vi "PCA9525 - 24V.vi"(8 "error in (no error)":errorcluster, 11 "handle":u64 format="%x") -> (0 "error out":errorcluster, 2 "buffer":u8[](array[numeric]), 3 "handle 2":u64)   [LabVIEW 2024]
uses:
  I2C/libmpsse.dll
  I2C/libMPSSE-I2C.lvlib
panel:
  out "sizeTransferred 2":u32
  out "p/f4":bool
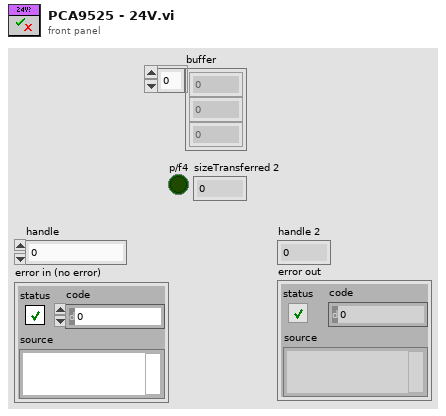
[diagram p1: front panel]
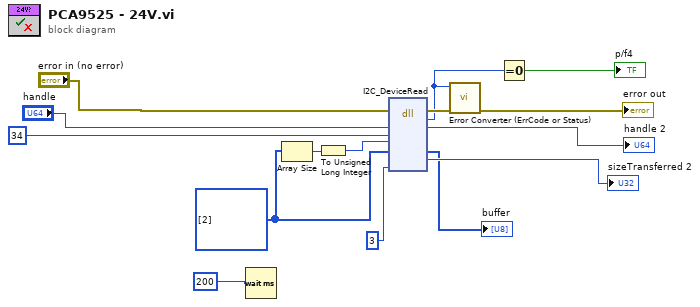
[diagram p0: block diagram]
diagram:
  w7 = u8[] [2] ("*buffer 3")
  n1 = Wait (ms)(milliseconds to wait=u32 200) -> ()  [unwired: 1 out]
  n2 = Array Size(array=w7) -> (size(s)=w6:i32)
  n3 = To Unsigned Long Integer(number=w6) -> (unsigned 32bit integer=w8:u32)
  n4 = dll-call lib="C:/Sandbox/sm_6576_001_RIB_Sequencer/I2C/libmpsse.dll" fn="I2C_DeviceRead"(error in="error in (no error)", "handle"="handle", "deviceAddress"=u8 34, "sizeToTransfer"=w8, "buffer"=w7, "options"=u32 3) -> (error out=w4:errorcluster, "return type"=w2:u64, "handle"=→"handle 2":u64, "buffer"=→"buffer":u8[], "sizeTransferred"=→"sizeTransferred 2":u32)  [unwired: 6 in, 1 out]
  n5 = call "Error Converter (ErrCode or Status).vi"("error in (no error)"=w4, "error code"=w2) -> ("error out"=→"error out":errorcluster)  [unwired: 9 in]
  n6 = Equal To 0?(x=w2) -> (x = 0?=→"p/f4":bool)
